vi "ITX to HDF5.vi"(8 "error in (no error)":errorcluster, 10 "file (use dialog)":path=path "P:/sample/GaAs/GaAs quantum dots/2008/PL Map/A1 735/060731ASBA_A1_6.0.itx", 11 "LV to ITX.lvclass":refnum<class "LV to ITX.lvclass">) -> (0 "error out":errorcluster, 3 "LV to ITX.lvclass":refnum<class "LV to ITX.lvclass">)   [LabVIEW 2016, in "LV to ITX.lvclass"]
uses:
  LV to ITX.lvclass
  LV to ITX.lvclass/LV to ITX.ctl
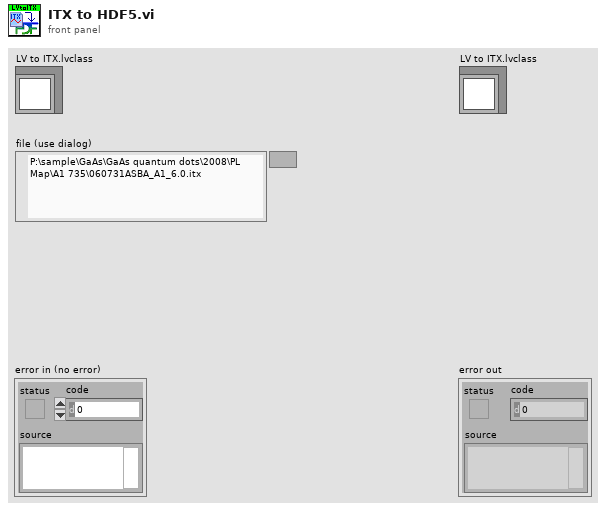
[diagram p1: front panel]
types:
  T1 = typedef "LV to ITX.lvclass/Dictionary--cluster.ctl" = cluster{"key":string, "value":variant}
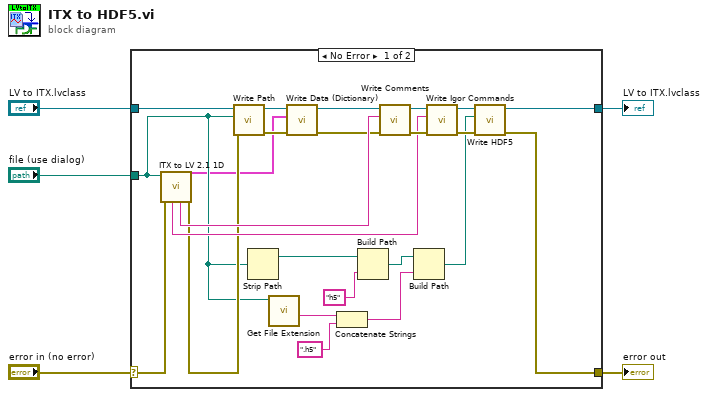
[diagram p0: block diagram]
diagram:
  n1 = case shown="No Error" "error in (no error)" {
    selector: "error in (no error)" -> [w29 w31]
    tunnel: [w18 w31] -> w4
    tunnel: [w17 w30] -> w2
    tunnel: "LV to ITX.lvclass" -> [w27 w30]
    tunnel: "file (use dialog)" -> [w14 _]
    frame No Error {
      n2 = call "ITX to LV 2.1 1D.vi"("error in"=w29, "file (use dialog)"=w14) -> ("error out"=w19:errorcluster, "Data (Dictionary)"=w8:T1[], "Notes"=w28:string, "Commands"=w22:string)  [unwired: 4 in, 2 out]
      n3 = call "Write Path.vi"("error in (no error)"=w19, "Path"=w14, "LVtoITX in"=w27) -> ("error out"=w25:errorcluster, "LVtoITX out"=w26:refnum<class "LV to ITX.lvclass">)  [unwired: 7 in]
      n4 = Strip Path(path=w14) -> (stripped path=w9:path)  [unwired: 1 out]
      n5 = call <vilib>:"Get File Extension.vi"("file"=w14) -> ("filename without extension"=w16:string)  [unwired: 6 in, 4 out]
      n6 = call "Write Data (Dictionary).vi"("error in (no error)"=w25, "Data (Dictionary)"=w8, "LVtoITX in"=w26) -> ("error out"=w7:errorcluster, "LVtoITX out"=w6:refnum<class "LV to ITX.lvclass">)  [unwired: 7 in]
      n7 = Concatenate Strings(w16, ".h5" ("string")) -> (w15:string)
      n8 = Build Path(base path=w9, name or relative path="h5" ("string")) -> (appended path=w10:path)
      n9 = call "Write Comments.vi"("error in (no error)"=w7, "Comments"=w28, "LVtoITX in"=w6) -> ("error out"=w23:errorcluster, "LVtoITX out"=w24:refnum<class "LV to ITX.lvclass">)  [unwired: 7 in]
      n10 = Build Path(base path=w10, name or relative path=w15) -> (appended path=w13:path)
      n11 = call "Write Igor Commands.vi"("error in (no error)"=w23, "Igor Commands"=w22, "LVtoITX in"=w24) -> ("error out"=w20:errorcluster, "LVtoITX out"=w21:refnum<class "LV to ITX.lvclass">)  [unwired: 7 in]
      n12 = call "Write HDF5.vi"("error in (no error)"=w20, "path"=w13, "LV to ITX.lvclass"=w21) -> ("error out"=w18:errorcluster, "LV to ITX.lvclass"=w17:refnum<class "LV to ITX.lvclass">)  [unwired: 7 in]
    }
    frame Error {
    }
  }
  "error out" <- w4
  "LV to ITX.lvclass" <- w2
